vi "write_attributes.vi"(8 "error in (no error)":errorcluster, 10 "attributes":T1, 11 "BernoulliNB in":refnum<class "BernoulliNB.lvclass">) -> (0 "error out":errorcluster, 3 "BernoulliNB out":refnum<class "BernoulliNB.lvclass">)   [LabVIEW 2020, in "BernoulliNB.lvclass"]
uses:
  BernoulliNB.lvclass
  Controls/bernoulliNB_attributes.ctl
  BernoulliNB.lvclass/BernoulliNB.ctl
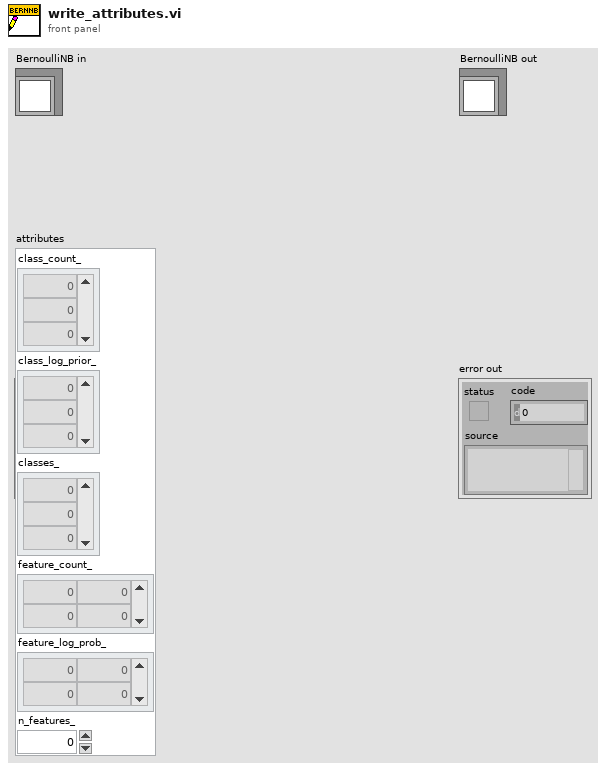
[diagram p1: front panel]
types:
  T1 = typedef "bernoulliNB_attributes.ctl" = cluster{"class_count_":dbl[], "class_log_prior_":dbl[], "classes_":dbl[], "feature_count_":dbl[][], "feature_log_prob_":dbl[][], "n_features_":dbl}
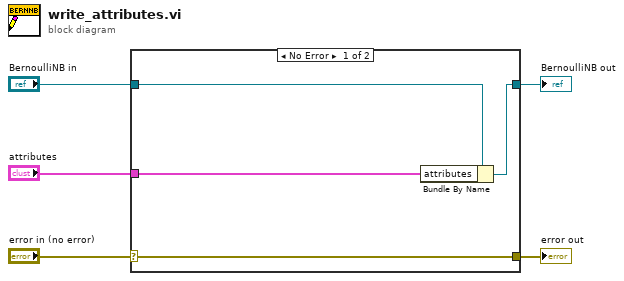
[diagram p0: block diagram]
diagram:
  n1 = case shown="No Error" "error in (no error)" {
    selector: "error in (no error)" -> [w9 w10]
    tunnel: [w9 w10] -> w4
    tunnel: [w7 w11] -> w2
    tunnel: "BernoulliNB in" -> [w8 w11]
    tunnel: "attributes" -> [w6 _]
    frame No Error {
      n2 = Bundle By Name(cluster=w8, "attributes"=w6) -> (w7:refnum<class "BernoulliNB.lvclass">)
    }
    frame Error {
    }
  }
  "error out" <- w4
  "BernoulliNB out" <- w2
